vi "Initialize.vi"(8 "error in (no error)":errorcluster, 11 "Protocol in":refnum<class "Protocol.lvclass">) -> (0 "error out":errorcluster, 3 "Protocol out":refnum<class "Protocol.lvclass">)   [LabVIEW 2020, in "CSM-FileSync.lvlib" / "Protocol.lvclass"]
uses:
  Protocol.lvclass
  Protocol.lvclass/Protocol.ctl
  <userlib>/_NEVSTOP/Communicable State Machine(CSM)/addons/Logger/CSM File Logger.lvlib
  <vilib>/NI/Tools/String/Tools_String.lvlib
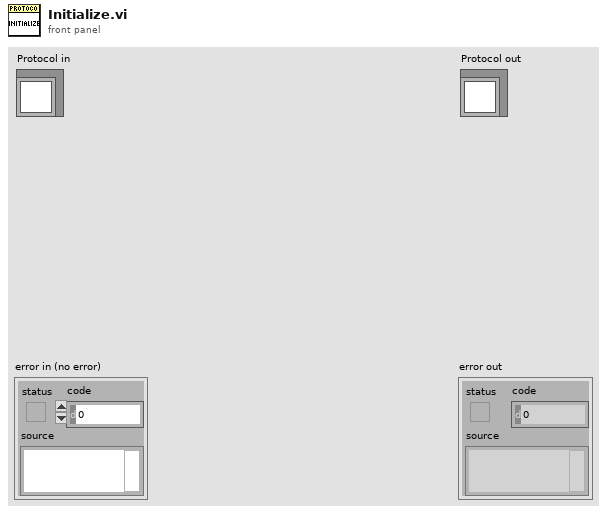
[diagram p1: front panel]
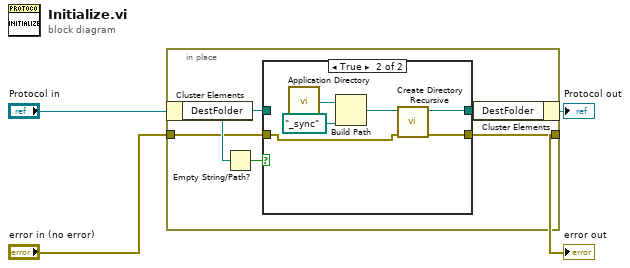
[diagram p0: block diagram]
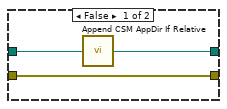
[diagram p2: hidden frame]
diagram:
  n1 = in-place {
    in-place-border: [w6] -> w2
    in-place-border: "error in (no error)" -> [w5]
    n2 = in-place-cluster #1("Protocol in") -> ("DestFolder"=w7:path)
    n3 = Empty String/Path?(string/path=w7) -> (empty?=w9:bool)
    n4 = case shown="True" w9 {
      tunnel: [w11 w15] -> w8
      tunnel: w7 -> [w12 _]
      tunnel: [w10 w14] -> w6
      tunnel: w5 -> [w10 w13]
      frame False {
        n5 = call <userlib>:"Append CSM AppDir If Relative.vi"("Relative Path (.)"=w12) -> ("Application Directory (+ Relative)"=w11:path)  [unwired: 4 in]
      }
      frame True {
        n6 = call <vilib>:"Application Directory.vi"() -> ("Application Directory"=w18:path)
        n7 = Build Path(base path=w18, name or relative path=path "_sync") -> (appended path=w17:path)
        n8 = call <vilib>:"Create Directory Recursive.vi"("error in"=w13, "directory"=w17) -> ("error out"=w14:errorcluster, "directory copy"=w15:path)  [unwired: 4 in]
      }
    }
    n9 = in-place-cluster #1("DestFolder"=w8) -> (→"Protocol out":refnum<class "Protocol.lvclass">)
  }
  "error out" <- w2
